vi "um to steps.vi"(9 "axis (default = fine)":enum16{"fine", "coarse"}(ring), 10 "position (microns)":dbl[unit]) -> (2 "steps":dbl)   [LabVIEW 2023]
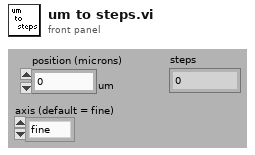
[diagram p1: front panel]
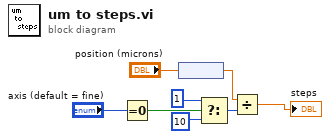
[diagram p0: block diagram]
diagram:
  n1 = Equal To 0?(x="axis (default = fine)") -> (x = 0?=w7:bool)
  n2 = node("position (microns)") -> (w2:dbl)
  n3 = Select(t=i8 1, s=w7, f=i8 10 ("y")) -> (s? t:f=w3:i8)
  n4 = Divide(x=w2, y=w3) -> (x/y=→"steps":dbl)
